vi "CMD_07T_SetRamp.vi"(8 "Ramp speed, K/min":dbl=5.0 min=0.1 max=10.0, 9 "Target, K":dbl=295.0 min=195.0 max=400.0, 11 "VISA resource name":refnum<visa-resource-name>) -> (3 "VISA resource name out":refnum<visa-resource-name>)   [LabVIEW 2013]
panel:
  out "unsigned 16bit integer":u16
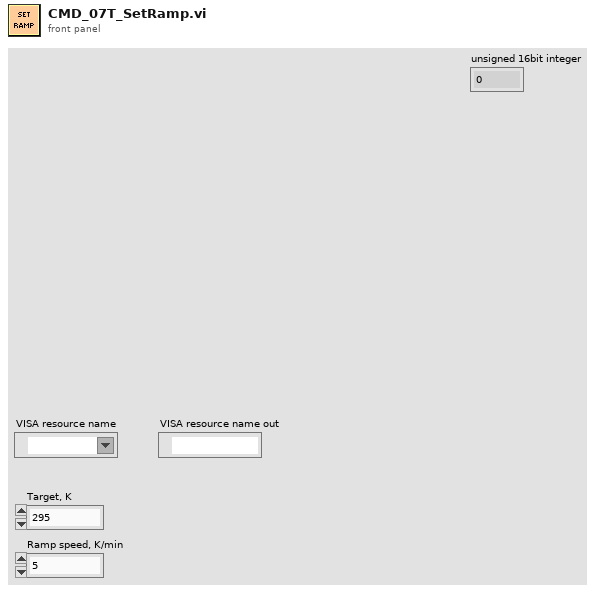
[diagram p1: front panel]
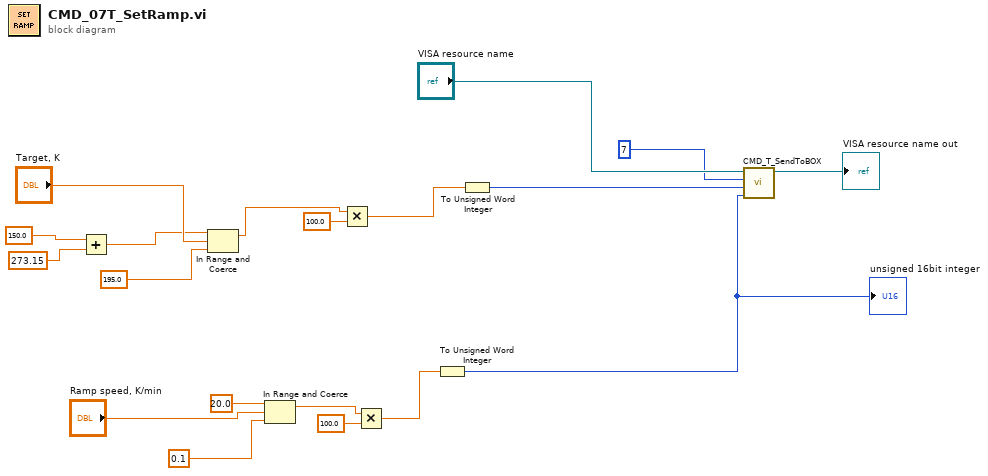
[diagram p0: block diagram]
diagram:
  n1 = Add(x=150.0, y=273.15) -> (x+y=w1:dbl)
  n2 = In Range and Coerce(upper limit=w1, x="Target, K", lower limit=195.0) -> (coerced(x)=w11:dbl)  [unwired: 1 out]
  n3 = In Range and Coerce(upper limit=20.0, x="Ramp speed, K/min", lower limit=0.1) -> (coerced(x)=w6:dbl)  [unwired: 1 out]
  n4 = Multiply(x=w11, y=100.0) -> (x*y=w15:dbl)
  n5 = Multiply(x=w6, y=100.0) -> (x*y=w5:dbl)
  n6 = To Unsigned Word Integer(number=w5) -> (unsigned 16bit integer=w4:u16)
  "unsigned 16bit integer" <- w4
  n7 = To Unsigned Word Integer(number=w15) -> (unsigned 16bit integer=w17:u16)
  n8 = call "CMD_T_SendToBOX.vi"("arg2"=w4, "arg1"=w17, "CMD"=i8 7, "VISA resource name"="VISA resource name") -> ("VISA resource name out"=→"VISA resource name out":refnum<visa-resource-name>)  [unwired: 7 in]
